vi "Create Serial Master.vi"(4 "flow control (none)":u16(ring) items=["None", "XON/XOFF", "RTS/CTS", "XON/XOFF & RTS/CTS", "DTR/DSR", "XON/XOFF & DTR/DSR"], 6 "parity (even)":u16(ring)=2 items=["None", "Odd", "Even", "Mark", "Space"], 7 "serial type":enum16{"RTU", "ASCII"}(ring), 8 "error in":errorcluster, 9 "Stop Bits(1.0)":u16(ring)=10 items=["1.0"=10, "1.5"=15, "2.0"=20], 10 "baud rate":u32=9600, 11 "VISA resource name":refnum<visa-resource-name>) -> (0 "error out":errorcluster, 3 "serial master instance":refnum<class "Modbus Master.lvclass">)   [LabVIEW 2013, in "Modbus Library - Advance.lvlib" / "API Main.lvlib"]
doc: "Creates a standard serial master. The transmission data unit used by the device is defined by the <B>serial type</B> input."
uses:
  API Main.lvlib
  Master/Modbus Master.lvclass
  Transmission Data Unit/RTU/RTU Data Unit.lvclass
  Transmission Data Unit/RTU/RTU Data Unit.lvclass/RTU Data Unit.ctl
  Transmission Data Unit/ASCII/ASCII Data Unit.lvclass
  Master Function Definition/Master Function Definition.lvclass
  Network Protocol/Network Master/Serial/Serial Master.lvclass
  Transmission Data Unit/Transmission Data Unit.lvclass/Transmission Data Unit.ctl
  Network Protocol/Network Master/Serial/Serial Master.lvclass/Serial Master.ctl
  Master/Modbus Master.lvclass/Modbus Master.ctl
  Modbus API.lvclass/Modbus API.ctl
  Network Protocol/Network Master/Serial/Write Serial Data Unit.vi
  Network Protocol/Network Master/Serial/Write Baud Rate.vi
  Network Protocol/Network Master/Serial/Write Parity.vi
  Network Protocol/Network Master/Serial/Write VISA resource name.vi
  Network Protocol/Network Master/Serial/Write Flow Control.vi
  Modbus API.lvclass
  Transmission Data Unit/Transmission Data Unit.lvclass
panel:
  # "disable parity disallowed by mbspec"
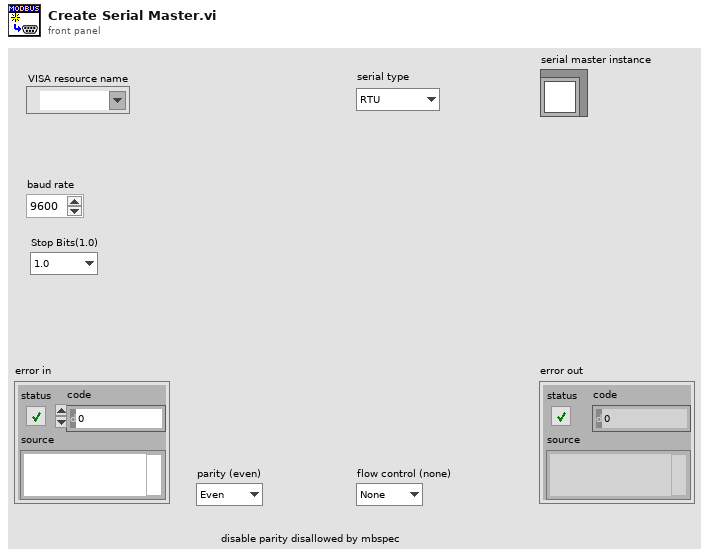
[diagram p1: front panel]
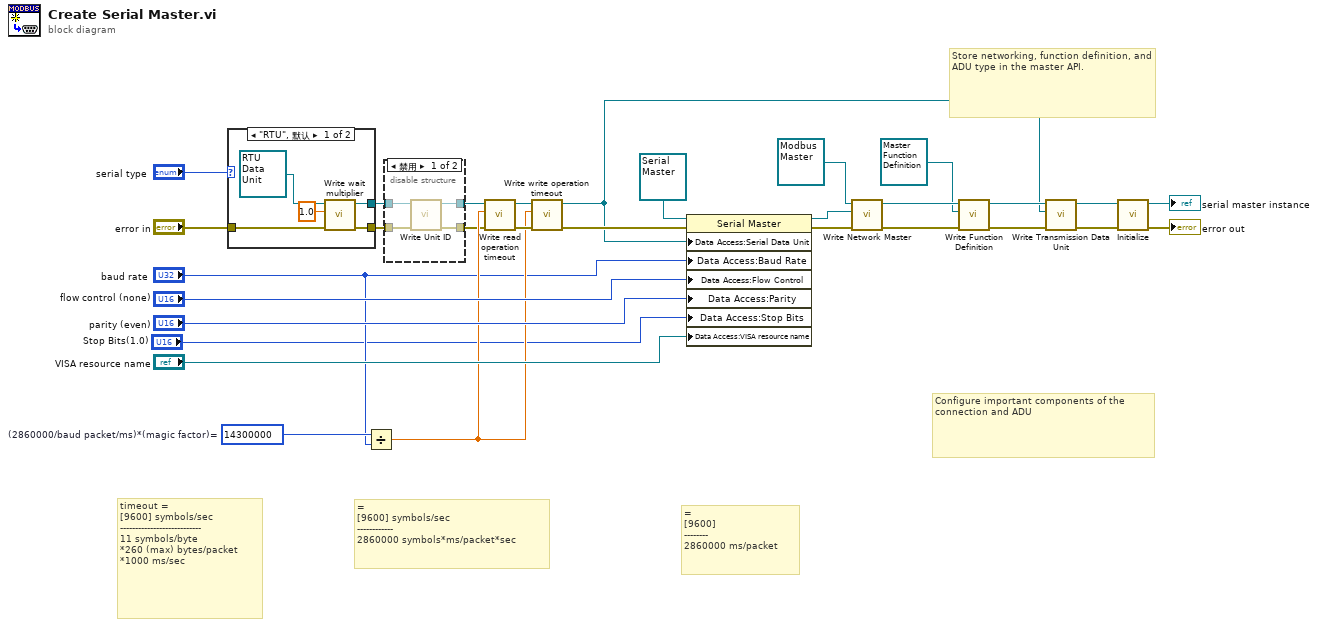
[diagram p0: block diagram]
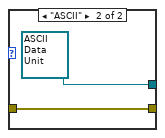
[diagram p3: hidden frame]
diagram:
  w13 = u32 14300000  # (2860000/baud packet/ms)*(magic factor)=
  # "=\n[9600]\n--------\n2860000 ms/packet"
  # "=\n[9600] symbols/sec\n------------\n2860000 symbols*ms/packet*sec"
  # "timeout =\n[9600] symbols/sec\n---------------------------\n11 symbols/byte\n*260 (max) bytes/packet\n*1000 ms/sec"
  # "Configure important components of the connection and ADU"
  # "Store networking, function definition, and ADU type in the master API."
  n1 = case shown="\"RTU\", 默认" "serial type" {
    tunnel: [w35 refnum<class "ASCII Data Unit.lvclass"> refnum ("ASCII Data Unit")] -> w1
    tunnel: "error in" -> [w33 w36]
    tunnel: [w34 w36] -> w2
    frame "RTU", Default {
      n2 = call "Write wait multiplier.vi"("error in (no error)"=w33, "wait multiplier"=sgl 1.0, "RTU Data Unit in"=refnum<class "RTU Data Unit.lvclass"> refnum ("RTU Data Unit")) -> ("error out"=w34:errorcluster, "RTU Data Unit out"=w35:refnum<class "RTU Data Unit.lvclass">)  [unwired: 7 in]
    }
    frame "ASCII" {
    }
  }
  n3 = Divide(x=w13, y="baud rate") -> (x/y=w8:dbl)
  n4 = disable-structure shown="禁用" {
    disable-tunnel: [w41 w43] -> w4
    disable-tunnel: [w40 w42] -> w3
    disable-tunnel: w2 -> [w39 w42]
    disable-tunnel: w1 -> [w38 w43]
    frame Disabled {
      n5 = call "Write Unit ID.vi"("error in"=w39, "transmission data unit in"=w38) -> ("error out"=w40:errorcluster, "transmission data unit out"=w41:refnum<class "Serial Data Unit.lvclass">)  [unwired: 8 in]
    }
    frame Enabled {
    }
  }
  n6 = call "Write read operation timeout.vi"("error in (no error)"=w3, "read operation timeout"=w8, "transmission data unit in"=w4) -> ("error out"=w11:errorcluster, "transmission data unit out"=w12:refnum<class "Serial Data Unit.lvclass">)  [unwired: 7 in]
  n7 = call "Write write operation timeout.vi"("error in (no error)"=w11, "write operation timeout"=w8, "transmission data unit in"=w12) -> ("error out"=w10:errorcluster, "transmission data unit out"=w9:refnum<class "Serial Data Unit.lvclass">)  [unwired: 7 in]
  n8 = property class="Serial Master"(reference=refnum<class "Serial Master.lvclass"> refnum ("Serial Master"), error in=w10, "Data Access:Serial Data Unit"=w9, "Data Access:Baud Rate"="baud rate", "Data Access:Flow Control"="flow control (none)", "Data Access:Parity"="parity (even)", "Data Access:Stop Bits"="Stop Bits(1.0)", "Data Access:VISA resource name"="VISA resource name") -> (reference out=w14:refnum<class "Serial Master.lvclass">, error out=w23:errorcluster)
  n9 = call "Write Network Master.vi"("error in"=w23, "network master"=w14, "Modbus master in"=refnum<class "Modbus Master.lvclass"> refnum ("Modbus Master")) -> ("error out"=w16:errorcluster, "Modbus master out"=w21:refnum<class "Modbus Master.lvclass">)  [unwired: 7 in]
  n10 = call "Write Function Definition.vi"("error in"=w16, "master function definition"=refnum<class "Master Function Definition.lvclass"> refnum ("Master Function Definition"), "Modbus master in"=w21) -> ("error out"=w17:errorcluster, "Modbus master out"=w20:refnum<class "Modbus Master.lvclass">)  [unwired: 7 in]
  n11 = call "Write Transmission Data Unit.vi"("error in"=w17, "transmission data unit"=w9, "Modbus instance in"=w20) -> ("error out"=w18:errorcluster, "Modbus instance out"=w19:refnum<class "Modbus Master.lvclass">)  [unwired: 7 in]
  n12 = call-dynamic "Initialize.vi"("error in"=w18, "Modbus master in"=w19) -> ("error out"=→"error out":errorcluster, "Modbus master out"=→"serial master instance":refnum<class "Modbus Master.lvclass">)  [unwired: 8 in]
